vi "PulseTrainGenerator.vi"(8 "Stop Button":bool, 11 "Channels Setup":T1(array[cluster])=[{"IP Address"="192.168.126.147", "DIO #"=0, "Frequency (Hz)"=200.0, "duty cycle (%)"=0.5, "Enable"=FALSE}, {"IP Address"="192.168.126.147", "DIO #"=1, "Frequency (Hz)"=90.0, "duty cycle (%)"=0.33, "Enable"=FALSE}]) -> ()   [LabVIEW 2015]
panel:
  in  "Startup Index":u16
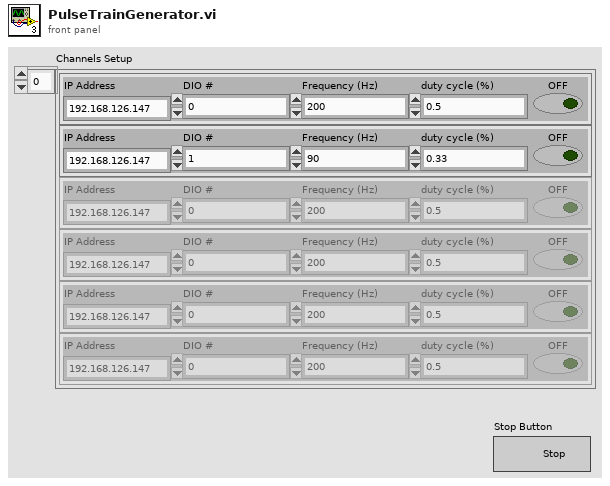
[diagram p1: front panel]
types:
  T1 = cluster{"IP Address":string, "DIO #":u16, "Frequency (Hz)":dbl, "duty cycle (%)":dbl, "Enable":bool}[]
  T2 = enum16{"Enable", "Disable", "Configure", "Configure and Run"}
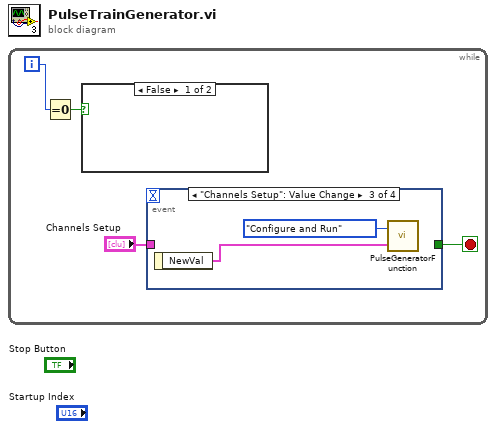
[diagram p0: block diagram]
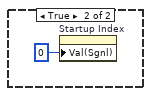
[diagram p2: hidden frame]
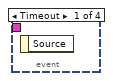
[diagram p3: hidden frame]
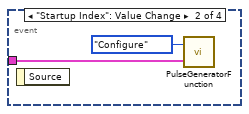
[diagram p4: hidden frame]
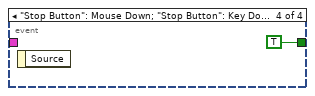
[diagram p5: hidden frame]
diagram:
  n1 = while {
    i -> [w3]
    stop <- w1 stop-if-true
    n2 = Equal To 0?(x=w3) -> (x = 0?=w2:bool)
    n3 = case shown="False" w2 {
      frame False {
      }
      frame True {
        n4 = property on="Startup Index" class="DigNum (strict)"("Val(Sgnl)"=u16 0 ("Value (Signaling)")) -> ()  [unwired: 2 in, 2 out]
      }
    }
    n5 = event shown="[2] \"Channels Setup\": Value Change" {
      selector: _ -> [_ _ _ _]
      dyn-events: _ -> [_ _ _ _]
      timeout: _ -> [_ _ _ _]
      tunnel: "Channels Setup" -> [_ w7 _ _]
      tunnel: [_ _ _ TRUE] -> w1
      event Timeout {
        n6 = event-data() -> ()  [unwired: 1 in, 1 out]
      }
      event "Startup Index": Value Change {
        n7 = event-data() -> ()  [unwired: 1 in, 1 out]
        n8 = call "PulseGeneratorFunction.vi"("Channels Setup"=w7, "Mode"=T2."Configure") -> ()  [unwired: 1 in]
      }
      event "Channels Setup": Value Change {
        n9 = event-data() -> ("NewVal"=w8:T1)  [unwired: 1 in]
        n10 = call "PulseGeneratorFunction.vi"("Channels Setup"=w8, "Mode"=T2."Configure and Run") -> ()  [unwired: 1 in]
      }
      event "Stop Button": Mouse Down; "Stop Button": Key Down {
        n11 = event-data() -> ()  [unwired: 1 in, 1 out]
      }
    }
  }
